vi "initialise.vi"(8 "error in (no error)":errorcluster, 11 "TrajectoryTS090820Circular2D in":refnum<class "TrajectoryTS090820Circular2D.lvclass">) -> (0 "error out":errorcluster, 3 "TrajectoryTS090820Circular2D out":refnum<class "TrajectoryTS090820Circular2D.lvclass">)   [LabVIEW 2010, in "TrajectoryTS090820Circular2D.lvclass"]
uses:
  TrajectoryTS090820Circular2D.lvclass
  common/enumerations/functional_global_action_enum.ctl
  common/enumerations/x_y_z_enumeration.ctl
  TrajectoryDL091126GenericVoxel/TrajectoryDL091126GenericVoxel/TrajectoryDL091126GenericVoxel.lvclass
panel:
  out "time needed [ms]":u32
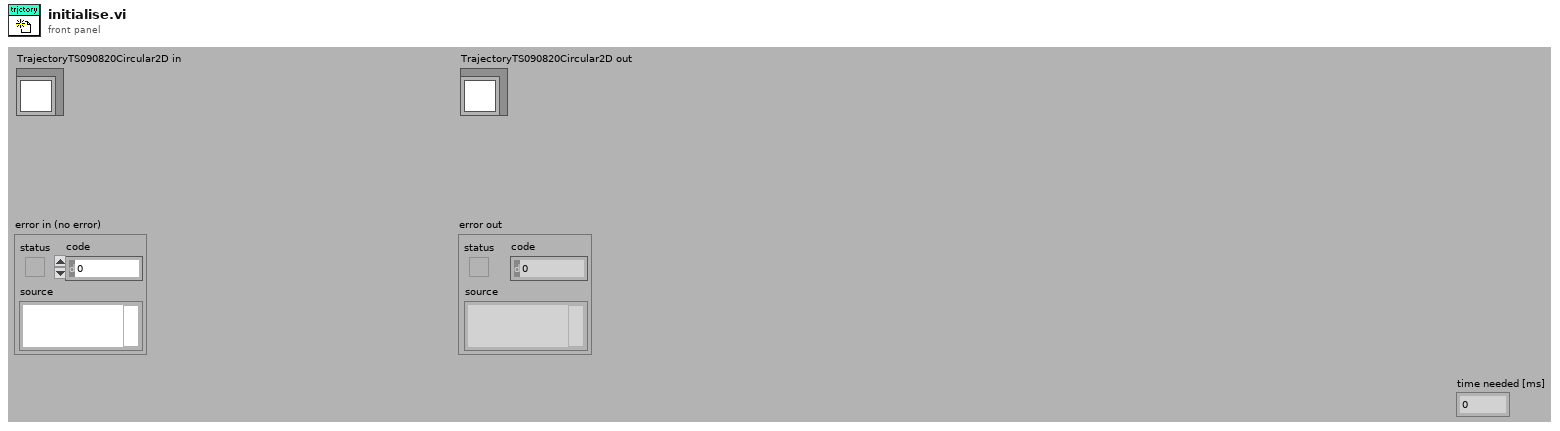
[diagram p1: front panel]
types:
  T1 = typedef "functional_global_action_enum.ctl" = enum16{"get", "set", "reset"}
  T2 = typedef "x_y_z_enumeration.ctl" = enum16{"x", "y", "z"}
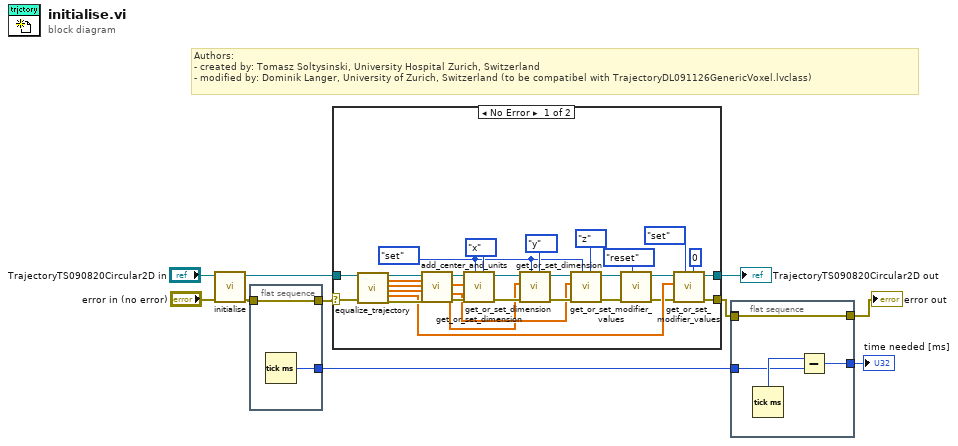
[diagram p0: block diagram]
diagram:
  # "Authors: \n- created by: Tomasz Soltysinski, University Hospital Zurich, Switzerland\n- modified by: Dominik Langer, University of Zurich, Switzerland (to be compatibel with TrajectoryDL091126GenericVoxel.lvclass)"
  n1 = call-parent "initialise.vi"("error in (no error)"="error in (no error)", "GenericTrajectory in"="TrajectoryTS090820Circular2D in") -> ("error out"=w6:errorcluster, "GenericTrajectory out"=w8:refnum<class "TrajectoryTS090820Circular2D.lvclass">)  [unwired: 8 in]
  n2 = flat-sequence {
    tunnel: w6 -> [w12]
    tunnel: [w12] -> w5
    tunnel: [w11] -> w2
    frame #0 {
      n3 = Tick Count (ms)() -> (millisecond timer value=w11:u32)
    }
  }
  n4 = case shown="No Error" w5 {
    selector: w5 -> [w28 w43]
    tunnel: [w34 w43] -> w4
    tunnel: [w33 w44] -> w7
    tunnel: w8 -> [w29 w44]
    frame No Error {
      w36 = functional_global_action_enum."set" ("action")
      n5 = call-dynamic "equalize_trajectory.vi"("TrajectoryTS090820Circular2D in"=w29, "error in (no error)"=w28) -> ("TrajectoryTS090820Circular2D out"=w27:refnum<class "TrajectoryTS090820Circular2D.lvclass">, "x trajectory"=w25:dbl[], "y trajectory"=w23:dbl[], "z trajectory"=w22:dbl[], "intensity"=w24:dbl[], "error out"=w26:errorcluster)  [unwired: 12 in]
      n6 = call-dynamic "add_center_and_units.vi"("TrajectoryTS090820Circular2D in"=w27, "x trajectory"=w25, "y trajectory"=w23, "z trajectory"=w22, "error in (no error)"=w26) -> ("TrajectoryTS090820Circular2D out"=w31:refnum<class "TrajectoryTS090820Circular2D.lvclass">, "x centered trajectory"=w14:dbl[unit][], "y centered trajectory"=w13:dbl[unit][], "z centered trajectory"=w15:dbl[unit][], "error out"=w30:errorcluster)  [unwired: 6 in]
      n7 = call-dynamic "get_or_set_dimension.vi"("dimension"=x_y_z_enumeration."x", "action"=w36, "error in (no error)"=w30, "pixel values in (single dimension)"=w14, "GenericTrajectory in"=w31) -> ("error out"=w39:errorcluster, "GenericTrajectory out"=w40:refnum<class "TrajectoryTS090820Circular2D.lvclass">)  [unwired: 4 in, 1 out]
      n8 = call-dynamic "get_or_set_dimension.vi"("dimension"=x_y_z_enumeration."y", "action"=w36, "error in (no error)"=w39, "pixel values in (single dimension)"=w13, "GenericTrajectory in"=w40) -> ("error out"=w38:errorcluster, "GenericTrajectory out"=w37:refnum<class "TrajectoryTS090820Circular2D.lvclass">)  [unwired: 4 in, 1 out]
      n9 = call-dynamic "get_or_set_dimension.vi"("dimension"=x_y_z_enumeration."z", "action"=w36, "error in (no error)"=w38, "pixel values in (single dimension)"=w15, "GenericTrajectory in"=w37) -> ("error out"=w20:errorcluster, "GenericTrajectory out"=w18:refnum<class "TrajectoryTS090820Circular2D.lvclass">)  [unwired: 4 in, 1 out]
      n10 = call-dynamic "get_or_set_modifier_values.vi"("action"=functional_global_action_enum."reset", "error in (no error)"=w20, "GenericTrajectory in"=w18) -> ("error out"=w19:errorcluster, "GenericTrajectory out"=w17:refnum<class "TrajectoryTS090820Circular2D.lvclass">)  [unwired: 6 in, 1 out]
      n11 = call-dynamic "get_or_set_modifier_values.vi"("modifier index"=0, "action"=functional_global_action_enum."set", "error in (no error)"=w19, "modifier values in"=w24, "GenericTrajectory in"=w17) -> ("error out"=w34:errorcluster, "GenericTrajectory out"=w33:refnum<class "TrajectoryTS090820Circular2D.lvclass">)  [unwired: 4 in, 1 out]
    }
    frame Error {
    }
  }
  "TrajectoryTS090820Circular2D out" <- w7
  n12 = flat-sequence {
    tunnel: w4 -> [w48]
    tunnel: [w48] -> _
    tunnel: [w48] -> w3
    tunnel: w2 -> [w46]
    tunnel: [w45] -> w1
    frame #0 {
      n13 = Tick Count (ms)() -> (millisecond timer value=w47:u32)
      n14 = Subtract(x=w47, y=w46) -> (x-y=w45:u32)
    }
  }
  "error out" <- w3
  "time needed [ms]" <- w1
